vi "Format Metadata.vi"(0 "SigMan in":refnum<class "SignalManager.lvclass">, 7 "Prefix":string, 11 "error in (no error)":errorcluster) -> (4 "SigMan out":refnum<class "SignalManager.lvclass">, 8 "String":string, 15 "error out":errorcluster)   [LabVIEW 2015, in "SignalManager.lvclass"]
uses:
  SignalManager.lvclass
  SignalManager.lvclass/SignalManager.ctl
  Channel/Channel.lvclass
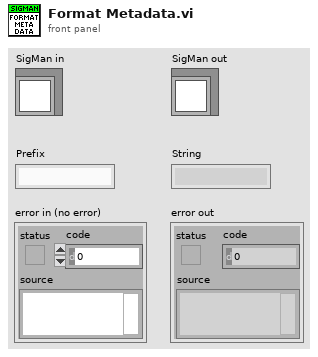
[diagram p1: front panel]
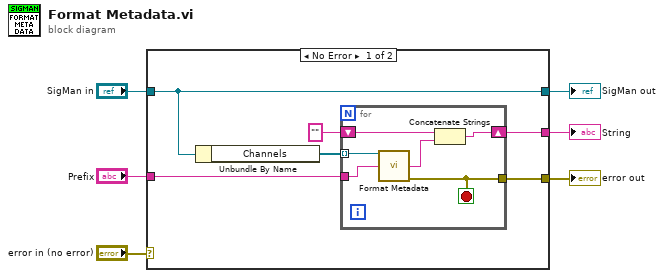
[diagram p0: block diagram]
diagram:
  n1 = case shown="No Error" "error in (no error)" {
    selector: "error in (no error)" -> [_ w20]
    tunnel: [w7 w20] -> w5
    tunnel: [w12 w19] -> w3
    tunnel: "SigMan in" -> [w12 w19]
    tunnel: "Prefix" -> [w9 _]
    tunnel: [w8 _] -> w1
    frame No Error {
      n2 = Unbundle By Name(w12) -> ("Channels"=w11:refnum<class "Channel.lvclass">[])
      n3 = for {
        tunnel: w11 -> [w18] mode=indexing
        shift-right: [w14] -> w8
        shift-left: "" -> [w16]
        tunnel: w9 -> [w17]
        tunnel: [w13] -> w7
        stop <- w13 stop-if-true
        n4 = call "Format Metadata.vi"("Channel in"=w18, "Prefix"=w17) -> ("String"=w15:string, "error out"=w13:errorcluster)  [unwired: 11 in, 1 out]
        n5 = Concatenate Strings(w16, w15) -> (w14:string)
      }
    }
    frame Error {
    }
  }
  "error out" <- w5
  "SigMan out" <- w3
  "String" <- w1
